vi "Read properMotion.vi"(8 "error in (no error)":errorcluster, 11 "FixedTarget in":refnum<class "FixedTarget.lvclass">) -> (0 "error out":errorcluster, 2 "ProperMotion.lvclass":refnum<class "ProperMotion.lvclass">, 3 "FixedTarget out":refnum<class "FixedTarget.lvclass">)   [LabVIEW 2022 SP3, in "TCSDataDefinitions.lvlib" / "TCSCommand.lvlib" / "TargetConfiguration.lvlib" / "Target.lvlib" / "FixedTarget.lvlib" / "FixedTarget.lvclass"]
uses:
  FixedTarget.lvclass
  ProperMotion/ProperMotion.lvclass
  FixedTarget.lvclass/FixedTarget.ctl
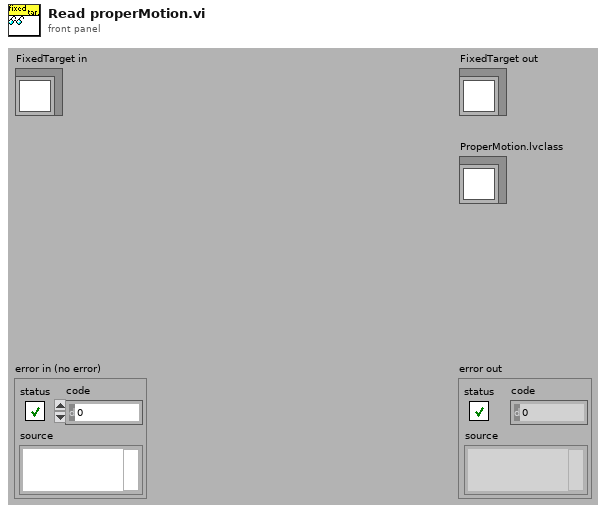
[diagram p1: front panel]
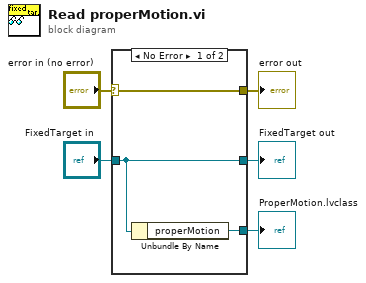
[diagram p0: block diagram]
diagram:
  n1 = case shown="No Error" "error in (no error)" {
    selector: "error in (no error)" -> [w8 w9]
    tunnel: [w8 w9] -> w4
    tunnel: [w7 w10] -> w2
    tunnel: "FixedTarget in" -> [w7 w10]
    tunnel: [w6 _] -> w1
    frame No Error {
      n2 = Unbundle By Name(w7) -> ("properMotion"=w6:refnum<class "ProperMotion.lvclass">)
    }
    frame Error {
    }
  }
  "error out" <- w4
  "FixedTarget out" <- w2
  "ProperMotion.lvclass" <- w1
